vi "Waveform to Data.vi"(11 "Data IN":waveform(dbl)[](array[waveform])) -> (3 "Data OUT":dbl[][](array[numeric]))   [LabVIEW 2019]
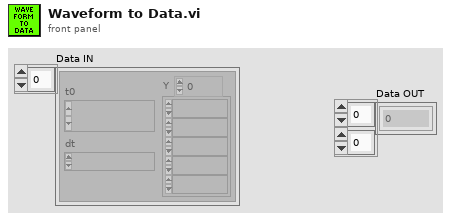
[diagram p1: front panel]
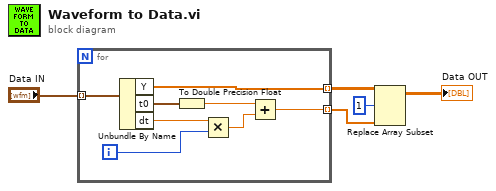
[diagram p0: block diagram]
diagram:
  n1 = for {
    tunnel: "Data IN" -> [w13] mode=indexing
    tunnel: [w7] -> w4 mode=indexing
    tunnel: [w6] -> w3 mode=indexing
    i -> [w11]
    n2 = Unbundle By Name(w13) -> ("Y"=w7:dbl[], "t0"=w10:timestamp, "dt"=w12:dbl)
    n3 = To Double Precision Float(number=w10) -> (double precision float=w8:dbl)
    n4 = Multiply(x=w12, y=w11) -> (x*y=w9:dbl)
    n5 = Add(x=w8, y=w9) -> (x+y=w6:dbl)
  }
  n6 = Replace Array Subset(array=w4, new element=w3, index (row)=1) -> (→"Data OUT":dbl[][])  [unwired: 1 in]
